vi "Increment File Name.vi"(1 "Full Path":path) -> (0 "New Path":path)   [LabVIEW 2013]
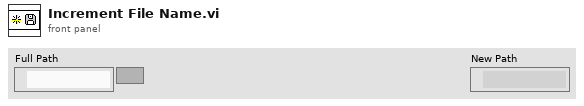
[diagram p1: front panel]
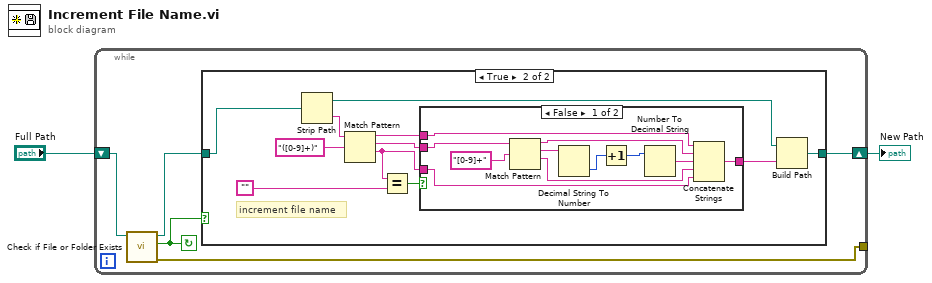
[diagram p0: block diagram]
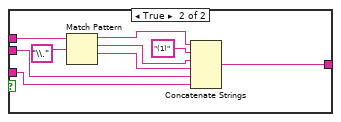
[diagram p3: hidden frame]
diagram:
  n1 = while {
    tunnel: [w4] -> _
    shift-right: [w7] -> w1
    shift-left: "Full Path" -> [w3]
    stop <- w5 continue-if-true
    n2 = call <vilib>:"Check if File or Folder Exists.vi"("path"=w3) -> ("error out"=w4:errorcluster, "file or folder exists?"=w5:bool, "dup path"=w6:path)  [unwired: 8 in]
    n3 = case shown="True" w5 {
      tunnel: w6 -> [w8 w19]
      tunnel: [w8 w18] -> w7
      frame False {
      }
      frame True {
        # "increment file name"
        n4 = Strip Path(path=w19) -> (stripped path=w12:path, name=w17:string)
        n5 = Match Pattern(string=w17, regular expression="([0-9]+)") -> (before substring=w13:string, match substring=w10:string, after substring=w9:string)  [unwired: 1 in, 1 out]
        n6 = Equal?(x=w9, y="") -> (x = y?=w14:bool)
        n7 = case shown="False" w14 {
          tunnel: w13 -> [w20 w39]
          tunnel: [w24 w31] -> w11
          tunnel: w10 -> [w30 w33]
          tunnel: w9 -> [w21 w32]
          frame False {
            n8 = Match Pattern(string=w30, regular expression="[0-9]+") -> (before substring=w23:string, match substring=w28:string, after substring=w22:string)  [unwired: 1 in, 1 out]
            n9 = Decimal String To Number(string=w28) -> (number=w27:i32)  [unwired: 2 in, 1 out]
            n10 = Increment(x=w27) -> (x+1=w26:i32)
            n11 = Number To Decimal String(number=w26) -> (decimal integer string=w25:string)  [unwired: 1 in]
            n12 = Concatenate Strings(w20, w23, w25, w22, w21) -> (w24:string)
          }
          frame True {
            n13 = Match Pattern(string=w39, regular expression="\\.") -> (before substring=w37:string, match substring=w35:string, after substring=w34:string)  [unwired: 1 in, 1 out]
            n14 = Concatenate Strings(w37, "(1)" ("string"), w35, w34, w33, w32) -> (w31:string)
          }
        }
        n15 = Build Path(base path=w12, name or relative path=w11) -> (appended path=w18:path)
      }
    }
  }
  "New Path" <- w1
